vi "DeleteFromArray.vi"(10 "Index":u32, 11 "StringArrayIn":string[](array[string])) -> (3 "StringArrayOut":string[](array[string]))   [LabVIEW 2014, in "ParametericRoutines.lvlib"]
uses:
  ParametericRoutines.lvlib
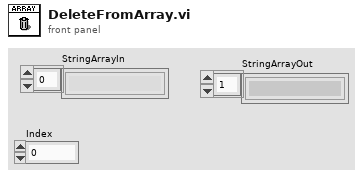
[diagram p1: front panel]
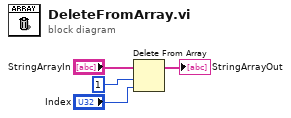
[diagram p0: block diagram]
diagram:
  n1 = Delete From Array(array="StringArrayIn", length=1, index="Index") -> (array with subset deleted=→"StringArrayOut":string[])  [unwired: 1 out]
